vi "Check Status.vi"(8 "error in (no error)":errorcluster, 11 "Pulse Gating System (HV supply) in":refnum<class "Pulse Gating System (HV supply).lvclass">) -> (0 "error out":errorcluster, 1 "Status":string, 2 "Ready?":bool, 3 "Pulse Gating System (HV supply) out":refnum<class "Pulse Gating System (HV supply).lvclass">)   [LabVIEW 2017, in "Pulse Gating System (HV supply).lvclass"]
doc: "(Dynamic) Check if the instrument is powered on and update its member fields with the instrument's current status. Optionally return a text status message."
uses:
  Pulse Gating System (HV supply).lvclass
  Pulse Gating System (HV supply).lvclass/Pulse Gating System (HV supply).ctl
  Utility Classes/Scannable/Scannable.lvclass
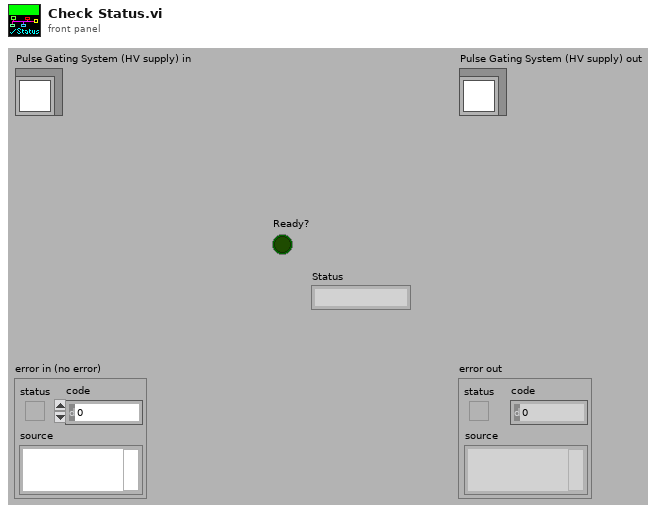
[diagram p1: front panel]
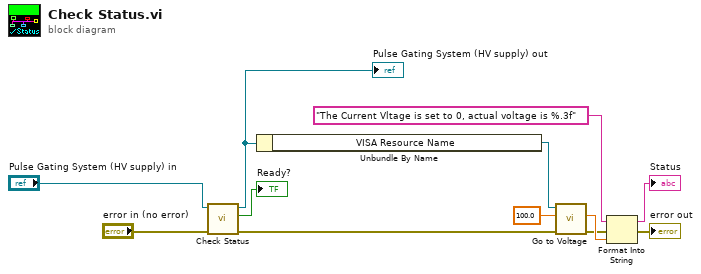
[diagram p0: block diagram]
diagram:
  n1 = call-parent "Check Status.vi"("error in (no error)"="error in (no error)", "Instrument in"="Pulse Gating System (HV supply) in") -> ("error out"=w12:errorcluster, "Ready?"=→"Ready?":bool, "Instrument out"=w1:refnum<class "Pulse Gating System (HV supply).lvclass">)  [unwired: 6 in, 1 out]
  "Pulse Gating System (HV supply) out" <- w1
  n2 = Unbundle By Name(w1) -> ("VISA Resource Name"=w8:refnum<visa-resource-name>)
  n3 = call "Go to Voltage.vi"("error in"=w12, "Set Voltage"=100.0, "VISA Resource Name"=w8) -> ("error out"=w9:errorcluster, "Actual Voltage"=w10:dbl)  [unwired: 6 in, 1 out]
  n4 = Format Into String(initial string="The Current Vltage is set to 0, actual voltage is %.3f", error in=w9, w10) -> (resulting string=→"Status":string, error out=→"error out":errorcluster)  [unwired: 1 in]
